vi "Speed Control.vi"(6 "Speed Up or Down?":bool, 9 "Min. speed":i32, 10 "Max. speed":i32, 11 "Ini. speed":i32) -> (1 "Speed out":i32)   [LabVIEW 2015]
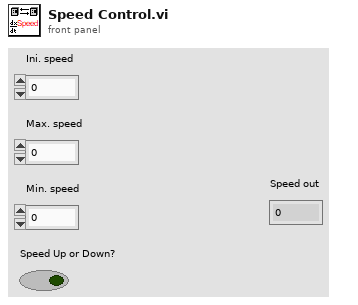
[diagram p1: front panel]
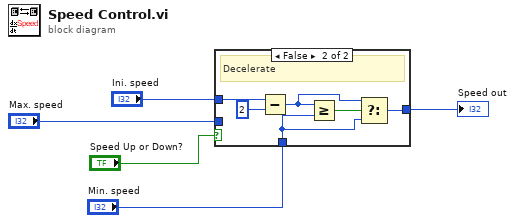
[diagram p0: block diagram]
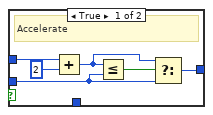
[diagram p2: hidden frame]
diagram:
  n1 = case shown="False" "Speed Up or Down?" {
    tunnel: "Max. speed" -> [w7 _]
    tunnel: "Ini. speed" -> [w10 w16]
    tunnel: [w6 w13] -> w5
    tunnel: "Min. speed" -> [_ w12]
    frame True {
      # "Accelerate"
      n2 = Add(x=w10, y=2) -> (x+y=w8:i32)
      n3 = Less Or Equal?(x=w8, y=w7) -> (x <= y?=w9:bool)
      n4 = Select(t=w8, s=w9, f=w7) -> (s? t:f=w6:i32)
    }
    frame False {
      # "Decelerate"
      n5 = Subtract(x=w16, y=2) -> (x-y=w14:i32)
      n6 = Greater Or Equal?(x=w14, y=w12) -> (x >= y?=w15:bool)
      n7 = Select(t=w14, s=w15, f=w12) -> (s? t:f=w13:i32)
    }
  }
  "Speed out" <- w5
